vi "Find Average Center.vi"(7 "Tray Number":i32, 9 "XYZTheta":dbl[](array[numeric]), 11 "Gantry In":refnum<k24>) -> (1 "XYZTheta Centers":dbl[][](array[numeric]), 3 "Gantry Out":refnum<k24>)   [LabVIEW 2021, in "Assembly Tray.lvclass"]
uses:
  Assembly Tray.lvclass
  Controller/Camera/Machine Vision.ctl
  C:/Program Files (x86)/Aerotech/A3200/LabVIEW/2010/Bin/Aerotech.A3200.dll
  Program Files (x86)/Aerotech/A3200/LabVIEW/2010/Bin/Aerotech.A3200.dll
  Find Tray.ctl
  Controller/Camera/Camera settings.ctl
  Controller/Camera/Image processing.ctl
  Controller/Camera/Material.ctl
  Controller/Camera/Camera.lvclass
  Controller/Motion/A3200/A3200.lvclass
  Controller/Motion/Motion.lvclass
panel:
  out "Syringe Area Recorded":bool
  out "All fiducials recorded":bool
  out "XY Graph":cluster{"X":dbl, "Y":dbl}[](graph)
  in  "Go to P6":bool
  in  "Go to P5":bool
  out "P5 XY":dbl[](array[numeric])
  out "P6 XY":dbl[](array[numeric])
  in  "Record P6":bool
  in  "Record P5":bool
  in  "Focus step size":dbl format="%#_13g"
  in  "number of focus steps":i32
  in  "Focus":bool
  out "Average Strength":dbl
  in  "Material":T1
  in  "Image processing":T2={"Brightness"=128.0, "Contrast"=45.0, "Gamma"=1.0471123} {"Brightness" scale=0.0..400.0; "Contrast" scale=0.0..90.0; "Gamma" scale=0.005..5.0}
  in  "Camera settings":T3={"Gamma"=1.6, "Gain"=0, "Sharpness"=0, "Contrast"=0.0, "Exposure"=0.0078125} {"Exposure" min=0.000244140625 max=0.5 scale=0.0002..0.5; "Contrast" min=0.0 max=1.0 scale=0.001..1.0; "Sharpness" min=0 max=2 step=1 scale=0.0..2.0; "Gain" min=0 max=100 step=1 scale=0.1..100.0; "Gamma" min=0.01 max=10.0 scale=0.01..10.0}
  in  "Override presets":bool
  out "Center":dbl[](array[numeric])
  out "Syringe Area":dbl[](array[numeric])
  in  "Go to Syringe Area":bool
  in  "Record Syringe Area":bool
  in  "Carrier Tray":T4
  in  "Position":bool=TRUE
  in  "Go to Center":bool
  in  "Joystick":bool
  in  "Record P2":bool
  in  "Record P3":bool
  in  "Record P1":bool
  in  "Record P4":bool
  out "P3 XY":dbl[](array[numeric])
  out "P4 XY":dbl[](array[numeric])
  out "P2 XY":dbl[](array[numeric])
  out "P1 XY":dbl[](array[numeric])
  in  "Go to P1":bool
  in  "Go to P2":bool
  in  "Go to P3":bool
  in  "Go to P4":bool
  out "Gantry":dbl[](array[numeric])
  out "Sum":dbl[](array[numeric])
  in  "Stop Program":bool
  out "Image":T5(plugin-control)
  out "Camera":dbl[](array[numeric])
  in  "Machine Vision":T6
  # "1"
  # "2"
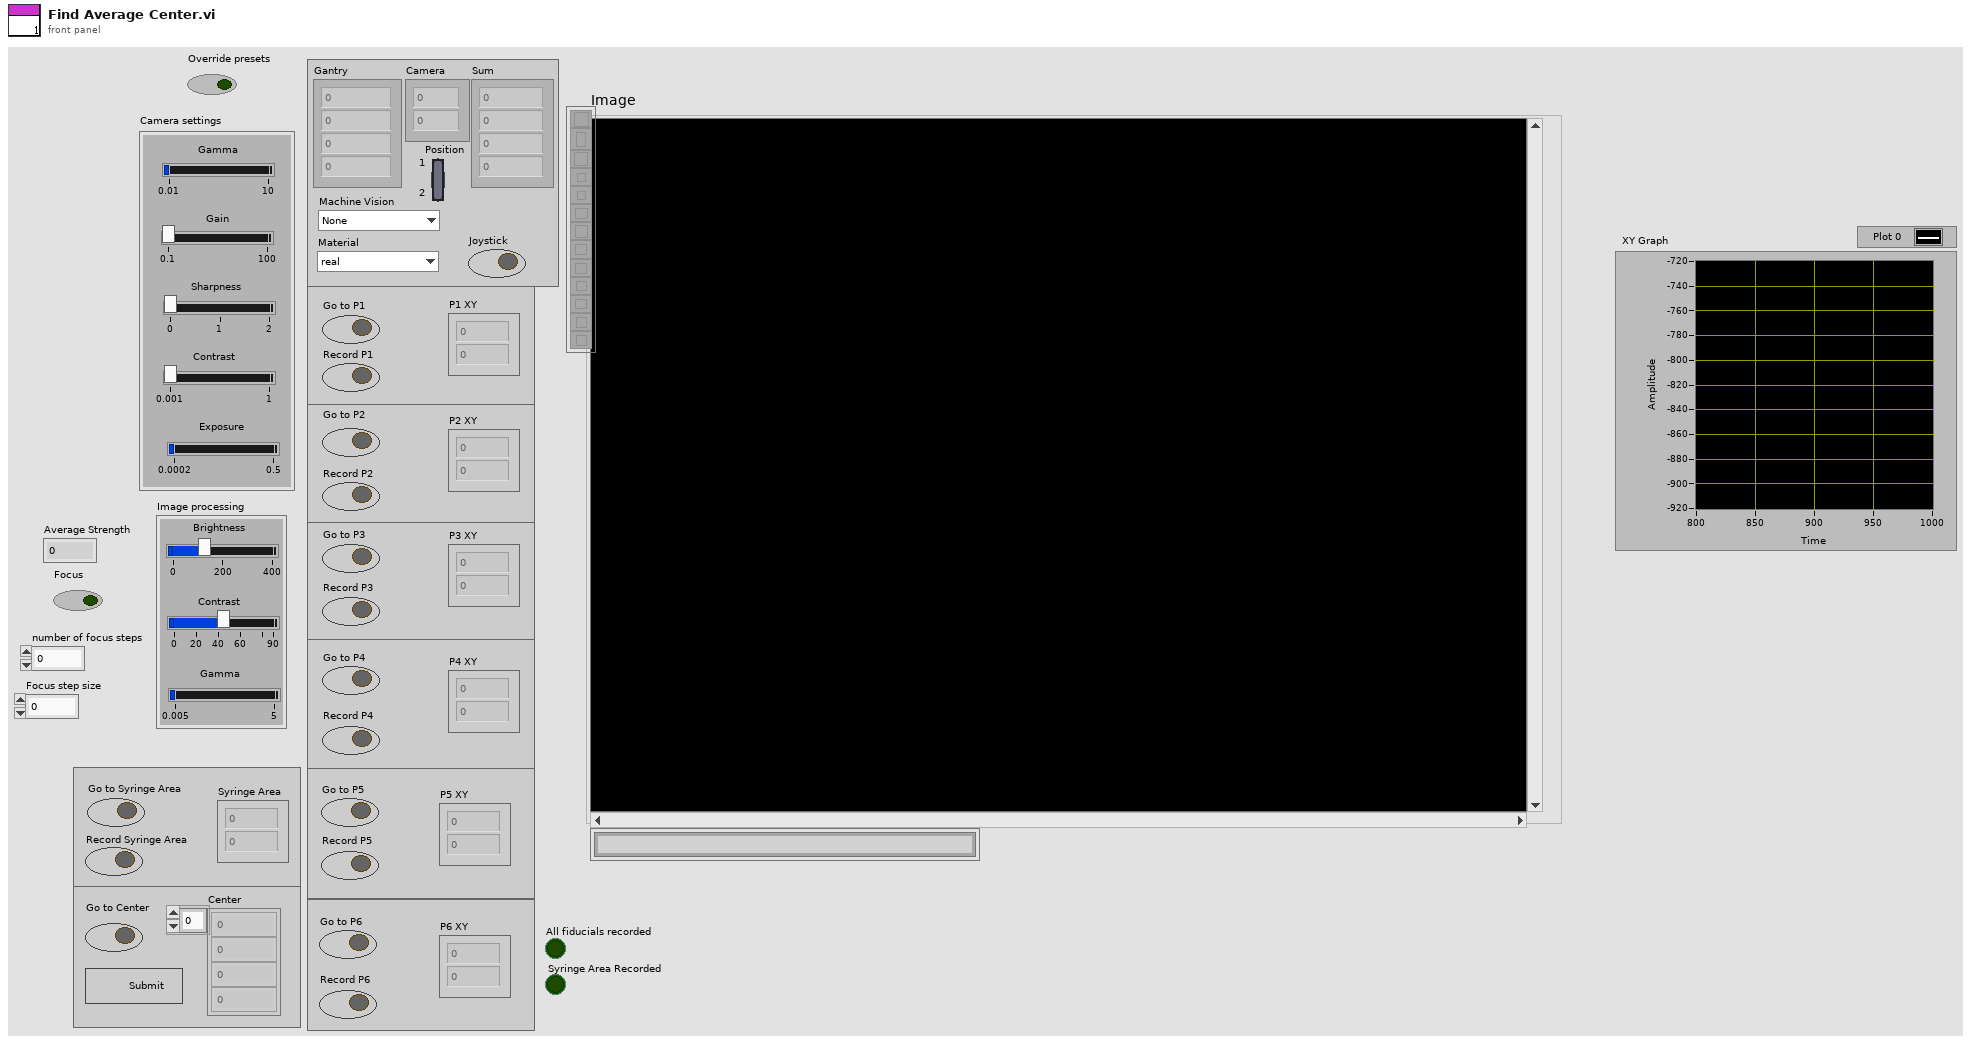
[diagram p1: front panel]
types:
  T1 = typedef "Camera.lvclass/Material.ctl" = enum16{"real", "dummy", "PETG"}
  T2 = typedef "Camera.lvclass/Image processing.ctl" = cluster{"Brightness":sgl, "Contrast":sgl, "Gamma":sgl}
  T3 = typedef "Camera.lvclass/Camera settings.ctl" = cluster{"Gamma":dbl, "Gain":i64, "Sharpness":i64, "Contrast":dbl, "Exposure":dbl}
  T4 = typedef "Assembly Tray.lvclass/Find Tray.ctl" = cluster{"Gantry Fiducials":dbl[], "Relative Coordinates":dbl[][], "Camera Fiducials":dbl[][], "XYZTheta Centers":dbl[][], "Workspace Center":dbl[], "Syringe Relative Coordinates":dbl[], "Gantry Region":dbl, "Fiducials":path, "New Fiducials":dbl[][], "Past Fiducials":dbl[][], "XYZTheta":dbl[], "Position":dbl}
  T5 = typedef "IMAQ Image.ctl" = refnum<image>
  T6 = typedef "Camera.lvclass/Machine Vision.ctl" = enum16{"None", "Tray Fiducials", "Sensor Fiducials", "HPK Silicon", "Partial Hexaboard", "Partial Hexaboard Test", "100um dot", "Hexaboard", "Corner (TL, BR)", "Corner (BL, TR)", "V3 Sensor Cross", "V3 Sensor Circle"}
  T7 = typedef "File Paths.ctl" = cluster{"Glue Pattern Folder":path, "Carrier Tray Folder":path, "Pick Up Tool Fixture Folder":path, "Components Folder":path, "Bellows Tool Offset.txt":path, "Pick Up Tool Offset.txt":path, "Dispense Tip Offset.txt":path, "Log Files":path, "Gantry Assembly Map.txt":path, "Syringe and offset map.txt":path}
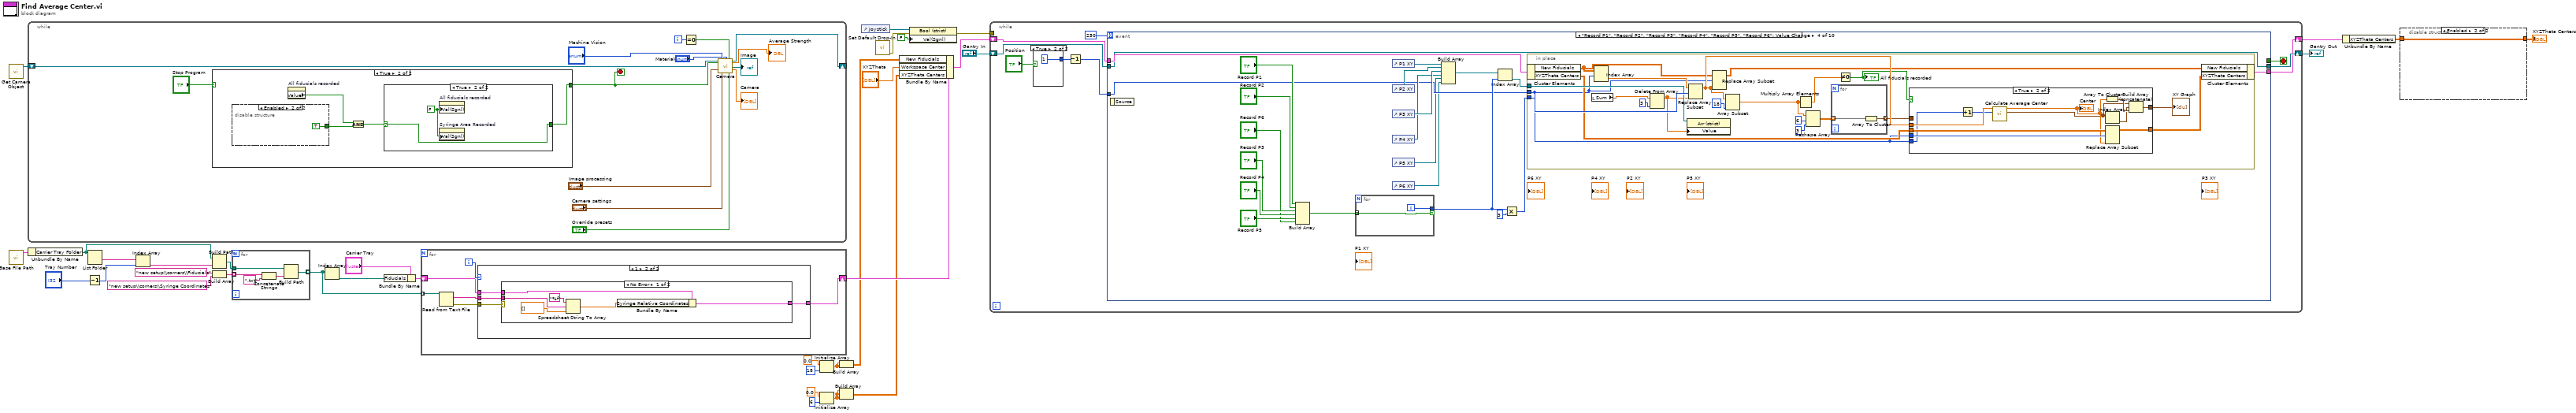
[diagram p0: block diagram]
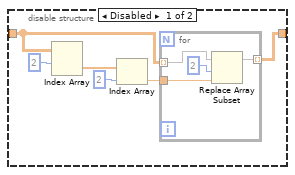
[diagram p2: hidden frame]
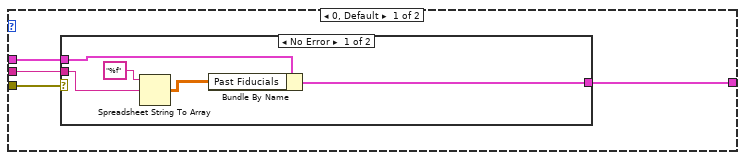
[diagram p3: hidden frame]
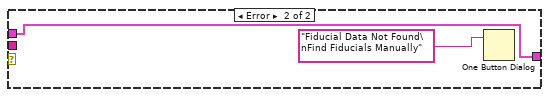
[diagram p4: hidden frame]
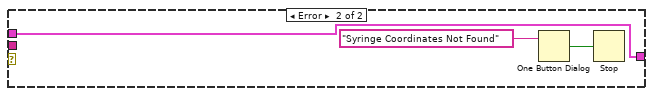
[diagram p5: hidden frame]
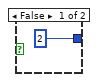
[diagram p6: hidden frame]
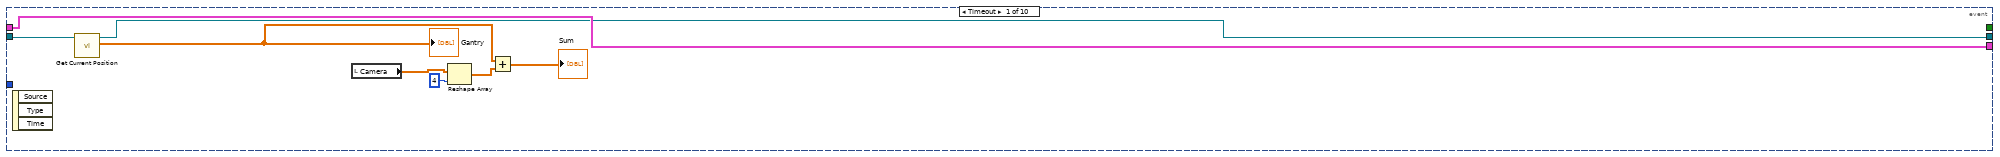
[diagram p7: hidden frame]
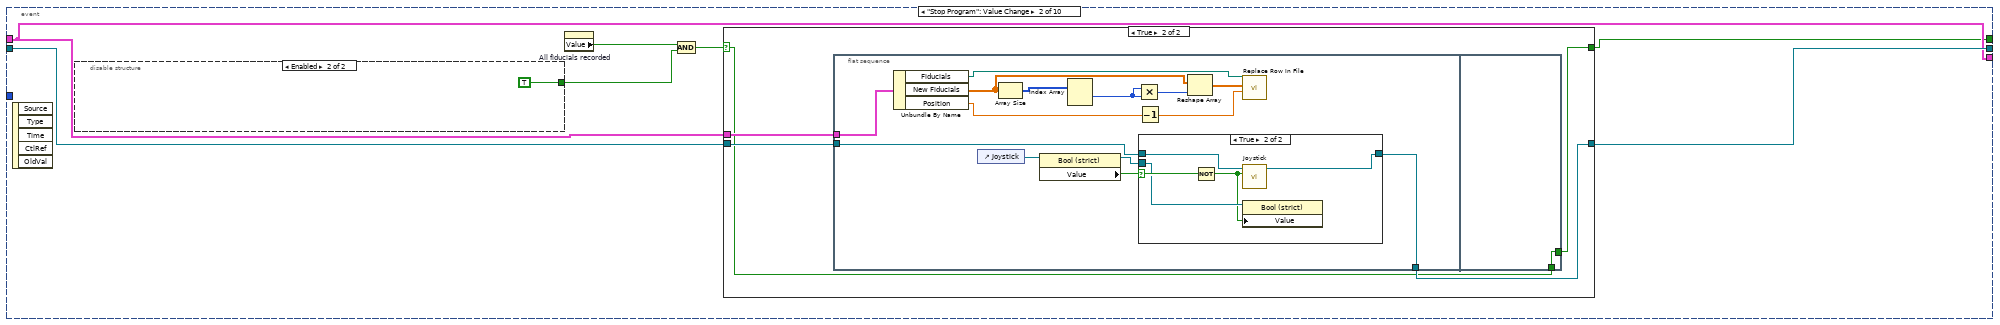
[diagram p8: hidden frame]
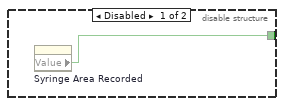
[diagram p9: hidden frame]
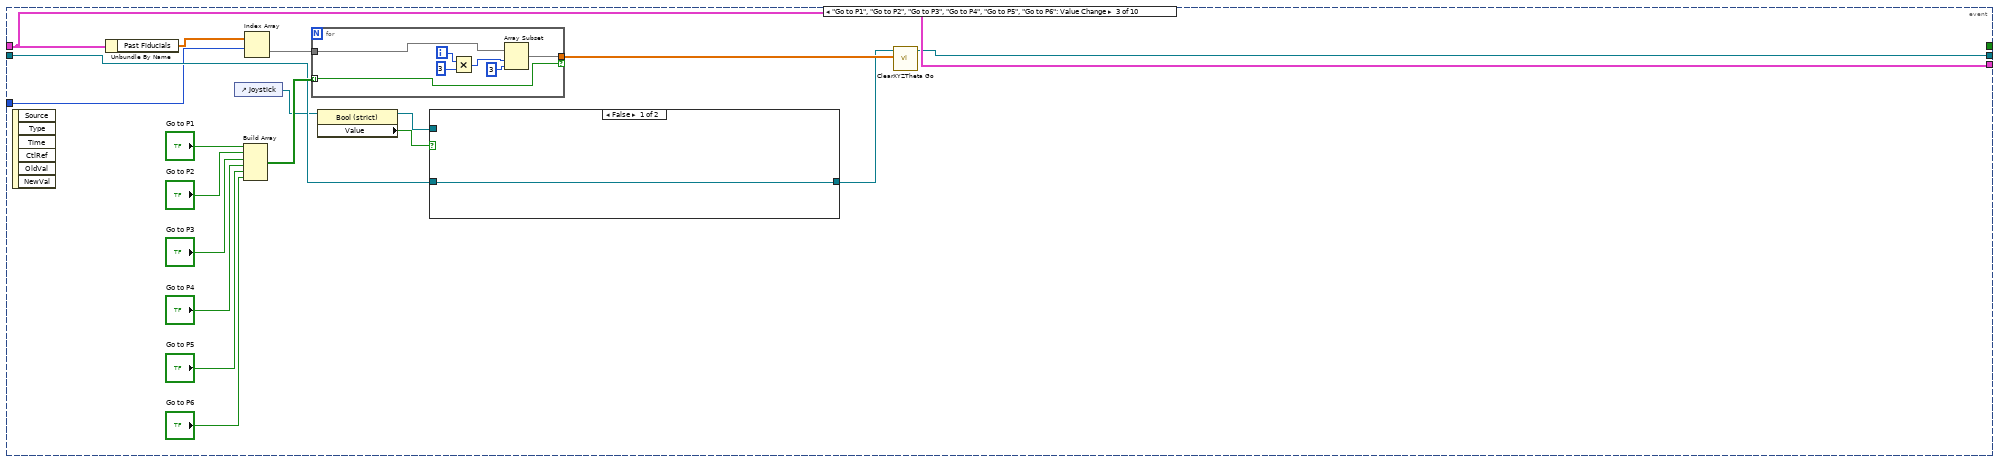
[diagram p12: hidden frame]
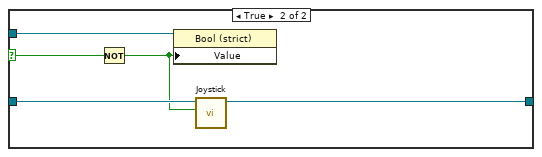
[diagram p13: hidden frame]
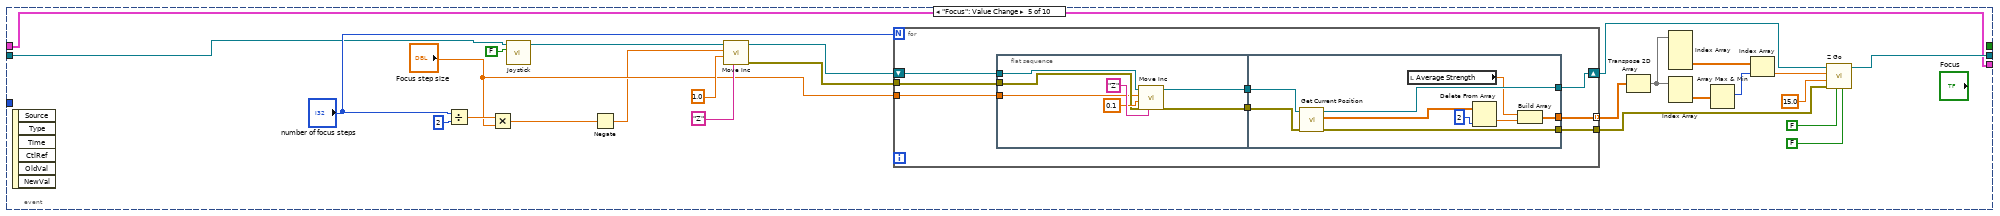
[diagram p15: hidden frame]
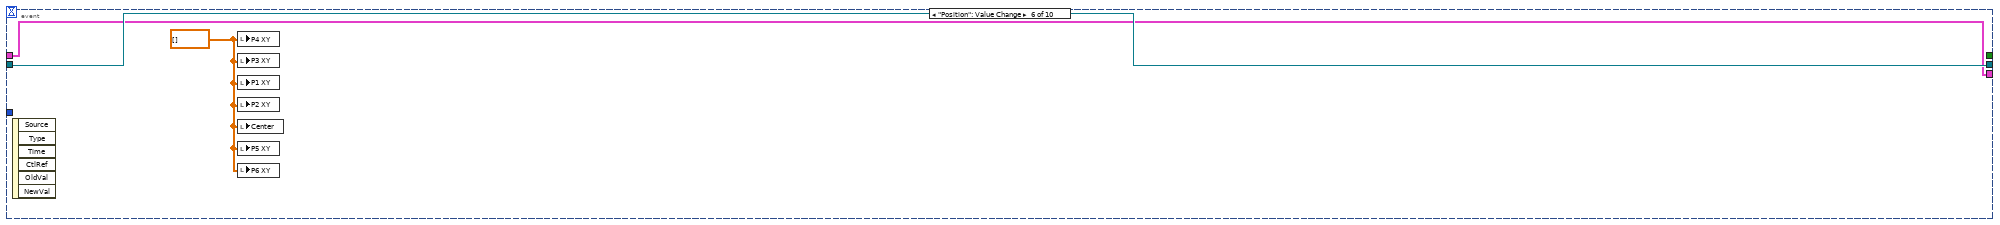
[diagram p16: hidden frame]
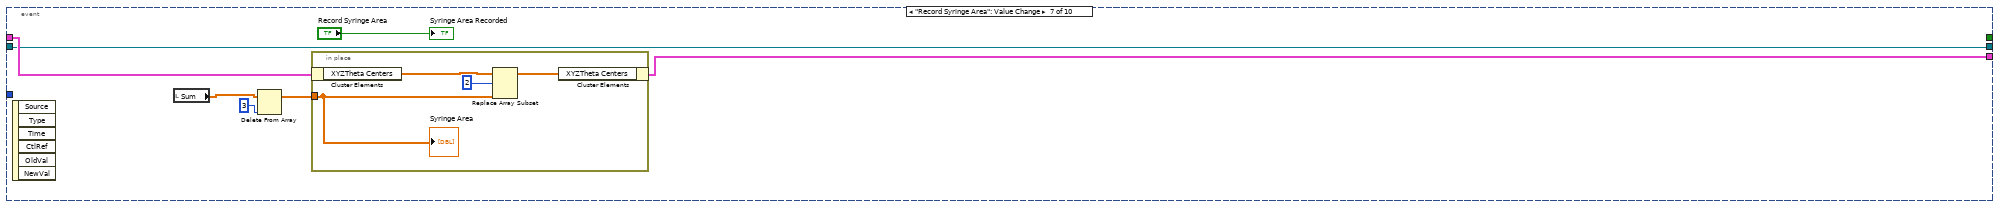
[diagram p17: hidden frame]
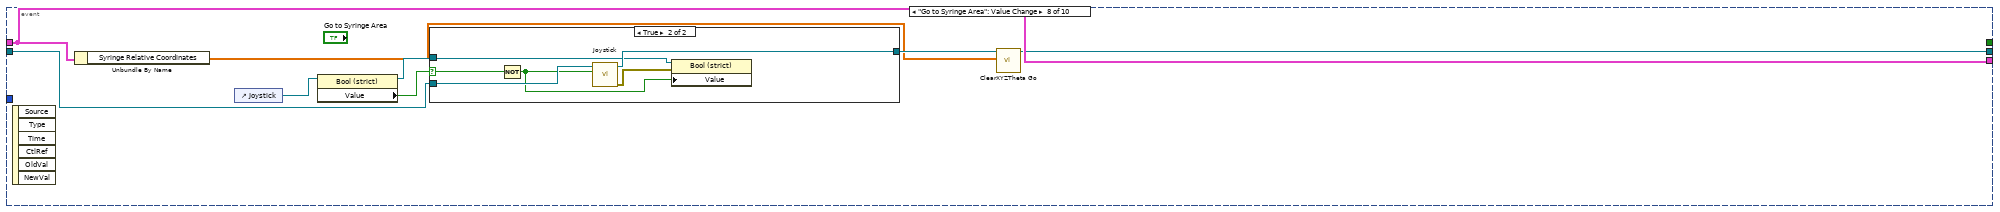
[diagram p18: hidden frame]
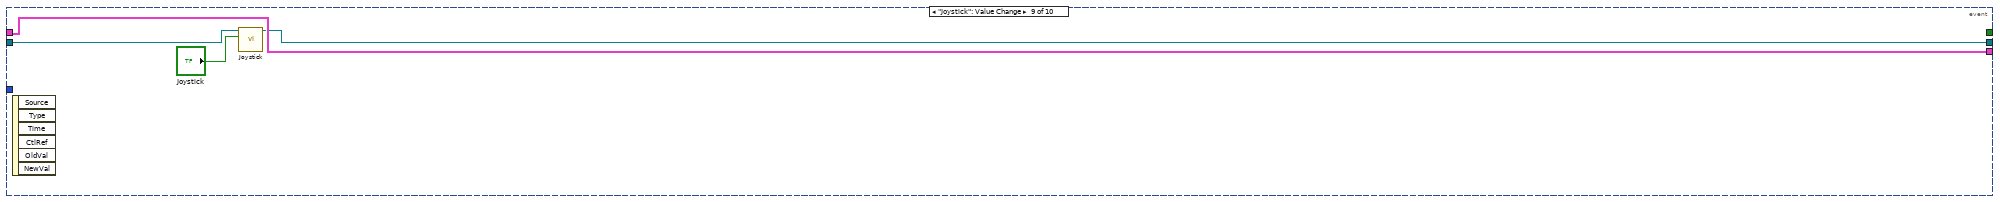
[diagram p20: hidden frame]
diagram:
  n1 = call "Get Camera Object.vi"() -> ("Camera out"=w3:refnum<class "Camera.lvclass">)  [unwired: 10 in, 1 out]
  n2 = call "Base File Path.vi"() -> ("Paths Out"=w19:T7)  [unwired: 11 in]
  n3 = while {
    shift-right: [w45] -> _
    shift-left: w3 -> [w49]
    i -> [w41]
    stop <- w36 stop-if-true
    n4 = case shown="True" "Stop Program" {
      selector: "Stop Program" -> [w50 _]
      tunnel: [w50 w51] -> w36
      frame False {
      }
      frame True {
        n5 = disable-structure shown="Enabled" {
          disable-tunnel: [w55 TRUE ("Value")] -> w53
          frame Disabled {
            n6 = property on="Syringe Area Recorded" class="Bool (strict)"() -> ("Value"=w55:bool)  [unwired: 2 in, 2 out]
          }
          frame Enabled {
          }
        }
        n7 = property on="All fiducials recorded" class="Bool (strict)"() -> ("Value"=w54:bool)  [unwired: 2 in, 2 out]
        n8 = And(x=w54, y=w53) -> (x .and. y?=w52:bool)
        n9 = case shown="True" w52 {
          selector: w52 -> [w58 w59]
          tunnel: [w58 w59] -> w51
          frame False {
            n10 = One Button Dialog(message="At least one fiducial or syringe loading area not recorded.") -> ()  [unwired: 1 in, 1 out]
          }
          frame True {
            w60 = FALSE ("Value (Signaling)")
            n11 = property on="All fiducials recorded" class="Bool (strict)"("Val(Sgnl)"=w60) -> ()  [unwired: 2 in, 2 out]
            n12 = property on="Syringe Area Recorded" class="Bool (strict)"("Val(Sgnl)"=w60) -> ()  [unwired: 2 in, 2 out]
          }
        }
      }
    }
    n13 = Equal To 0?(x=w41) -> (x = 0?=w40:bool)
    n14 = call "Camera.vi"("Camera in"=w49, "Stop"=w36, "BCG Image Processing"="Image processing", "Machine Vision"="Machine Vision", "Camera settings"="Camera settings", "Material"="Material", "Loop 0"=w40, "Override presets"="Override presets") -> ("Camera out"=w45:refnum<class "Camera.lvclass">, "Average Strength"=→"Average Strength":dbl, "Image"=→"Image":T5, "Camera"=→"Camera":dbl[])  [unwired: 5 in, 3 out]
  }
  n15 = Unbundle By Name(w19) -> ("Carrier Tray Folder"=w17:path)
  n16 = Decrement(x="Tray Number") -> (x-1=w18:i32)
  n17 = List Folder(path=w17) -> (folder names=w21:string[])  [unwired: 3 in, 3 out]
  n18 = Index Array(array=w21, index=w18) -> (element=w20:string)
  n19 = Build Path(base path=w17, name or relative path=w20) -> (appended path=w23:path)
  n20 = Build Array("new setup\\corners\\Fiducials" ("format string"), "new setup\\corners\\Syringe Coordinates" ("element")) -> (w22:string[])
  n21 = for {
    tunnel: w22 -> [w63] mode=indexing
    tunnel: w23 -> [w65]
    tunnel: [w64] -> w16 mode=indexing
    n22 = Concatenate Strings(w63, ".txt" ("string")) -> (w61:string)
    n23 = Build Path(base path=w65, name or relative path=w61) -> (appended path=w64:path)
  }
  n24 = Index Array(array=w16) -> (element=w2:path)  [unwired: 1 in]
  n25 = Bundle By Name(cluster="Carrier Tray", "Fiducials"=w2) -> (w25:T4)
  n26 = for {
    tunnel: w16 -> [w70] mode=indexing
    shift-right: [w66] -> w13
    shift-left: w25 -> [w67]
    i -> [w68]
    n27 = Read from Text File(file (use dialog)=w70) -> (text=w71:string, error out=w69:errorcluster)  [unwired: 3 in, 2 out]
    n28 = case shown="1" w68 {
      tunnel: w71 -> [w75 w84]
      tunnel: w69 -> [w74 w85]
      tunnel: w67 -> [w73 w86]
      tunnel: [w72 w83] -> w66
      frame 0, Default {
        n29 = case shown="No Error" w74 {
          tunnel: w75 -> [w79 _]
          tunnel: w73 -> [w77 w81]
          tunnel: [w78 w81] -> w72
          frame No Error {
            n30 = Spreadsheet String To Array(format string="%f", spreadsheet string=w79) -> (array=w76:dbl[][])  [unwired: 2 in]
            n31 = Bundle By Name(cluster=w77, "Past Fiducials"=w76) -> (w78:T4)
          }
          frame Error {
            n32 = One Button Dialog(message="Fiducial Data Not Found\nFind Fiducials Manually") -> ()  [unwired: 1 in, 1 out]
          }
        }
      }
      frame 1 {
        n33 = case shown="No Error" w85 {
          tunnel: w84 -> [w90 _]
          tunnel: [w88 w93] -> w83
          tunnel: w86 -> [w89 w93]
          frame No Error {
            n34 = Spreadsheet String To Array(format string="%f", spreadsheet string=w90, array type (2D Dbl)=dbl[] []) -> (array=w87:dbl[])  [unwired: 1 in]
            n35 = Bundle By Name(cluster=w89, "Syringe Relative Coordinates"=w87) -> (w88:T4)
          }
          frame Error {
            n36 = One Button Dialog(message="Syringe Coordinates Not Found") -> (true=w94:bool)  [unwired: 1 in]
            n37 = Stop(stop? (T)=w94) -> ()
          }
        }
      }
    }
  }
  n38 = Initialize Array(0.0 ("element"), 18 ("dimension size")) -> (w11:dbl[])
  n39 = Initialize Array(0.0 ("element"), 6 ("dimension size")) -> (w7:dbl[])
  n40 = Build Array(w11, w11) -> (w1:dbl[][])
  n41 = Build Array(w7, w7, w7) -> (w6:dbl[][])
  n42 = control-ref of="Joystick"() -> (w34:refnum<vi>)
  n43 = call "Set Default Drop-In.vi"() -> ("error out"=w28:errorcluster)  [unwired: 11 in]
  n44 = Bundle By Name(cluster=w13, "New Fiducials"=w1, "Workspace Center"="XYZTheta", "XYZTheta Centers"=w6) -> (w35:T4)
  n45 = property class="Bool (strict)"(reference=w34, error in=w28, "Val(Sgnl)"=FALSE) -> (error out=w32:errorcluster)  [unwired: 1 out]
  n46 = while {
    shift-right: [w97] -> w10
    shift-left: w35 -> [w104]
    tunnel: w32 -> [_]
    shift-right: [w101] -> w26
    shift-left: "Gantry In" -> [w102]
    stop <- w96 stop-if-true
    n47 = case shown="True" "Position" {
      tunnel: [2 1] -> w98
      frame False {
      }
      frame True {
      }
    }
    n48 = Decrement(x=w98) -> (x-1=w100:i32)
    n49 = event shown="[3] \"Record P1\", \"Record P2\", \"Record P3\", \"Record P4\", \"Record P5\", \"Record P6\": Value Change" {
      selector: _ -> [_ _ _ _ _ _ _ _ _ _]
      dyn-events: _ -> [_ _ _ _ _ _ _ _ _ _]
      timeout: 250 -> [_ _ _ _ _ _ _ _ _ _]
      tunnel: w104 -> [w113 w120 w163 w190 w245 w294 w302 w314 w325 w335]
      tunnel: [w113 w120 w163 w204 w245 w294 w301 w314 w325 w335] -> w97
      tunnel: w102 -> [w109 w119 w160 w183 w247 w295 w300 w313 w324 w331]
      tunnel: [w108 w121 w157 w183 w246 w295 w300 w308 w322 w329] -> w101
      tunnel: w100 -> [_ _ w154 w189 _ _ _ _ _ w327]
      tunnel: [_ w115 _ _ _ _ _ _ _ _] -> w96
      event Timeout {
        n50 = event-data() -> ()  [unwired: 1 in, 3 out]
        n51 = call "Get Current Position.vi"("Gantry In"=w109) -> ("XYZTheta Out"=w107:dbl[], "Gantry Out"=w108:refnum<k24>)  [unwired: 8 in, 1 out]
        "Gantry" <- w107
        n52 = local read "Camera"() -> (w112:dbl[])
        n53 = Reshape Array(w112, 4 ("dimension size")) -> (w110:dbl[])
        n54 = Add(x=w107, y=w110) -> (x+y=→"Sum":dbl[])
      }
      event "Stop Program": Value Change {
        n55 = event-data() -> ()  [unwired: 1 in, 5 out]
        n56 = disable-structure shown="Enabled" {
          disable-tunnel: [w122 TRUE ("Value")] -> w117
          frame Disabled {
            n57 = property on="Syringe Area Recorded" class="Bool (strict)"() -> ("Value"=w122:bool)  [unwired: 2 in, 2 out]
          }
          frame Enabled {
          }
        }
        n58 = property on="All fiducials recorded" class="Bool (strict)"() -> ("Value"=w118:bool)  [unwired: 2 in, 2 out]
        n59 = And(x=w118, y=w117) -> (x .and. y?=w116:bool)
        n60 = case shown="True" w116 {
          selector: w116 -> [w124 w127]
          tunnel: [w125 w130] -> w121
          tunnel: w120 -> [_ w129]
          tunnel: w119 -> [w125 w128]
          tunnel: [w124 w126] -> w115
          frame False {
          }
          frame True {
            n61 = flat-sequence {
              tunnel: [w144] -> w130
              tunnel: w129 -> [w135]
              tunnel: w128 -> [w131]
              tunnel: w127 -> [w151]
              tunnel: [w151] -> w126
              frame #0 {
                n62 = Unbundle By Name(w135) -> ("Fiducials"=w132:path, "New Fiducials"=w137:dbl[][], "Position"=w136:dbl)
                n63 = control-ref of="Joystick"() -> (w143:refnum<vi>)
                n64 = Array Size(array=w137) -> (size(s)=w138:i32[])
                n65 = property class="Bool (strict)"(reference=w143) -> (reference out=w142:refnum<vi>, "Value"=w141:bool)  [unwired: 1 in, 1 out]
                n66 = Index Array(array=w138) -> (element #1=w139:i32)  [unwired: 2 in, 1 out]
                n67 = Multiply(x=w139, y=w139) -> (x*y=w140:i32)
                n68 = Decrement(x=w136) -> (x-1=w133:dbl)
                n69 = case shown="True" w141 {
                  selector: w141 -> [_ w150]
                  tunnel: [w145 w148] -> w144
                  tunnel: w142 -> [_ w149]
                  tunnel: w131 -> [w145 w146]
                  frame False {
                  }
                  frame True {
                    n70 = Not(x=w150) -> (.not. x?=w147:bool)
                    n71 = call "Joystick.vi"("Joystick"=w147, "Gantry In"=w146) -> ("Gantry Out"=w148:refnum<k24>)  [unwired: 8 in, 1 out]
                    n72 = property class="Bool (strict)"(reference=w149, "Value"=w147) -> ()  [unwired: 1 in, 2 out]
                  }
                }
                n73 = Reshape Array(w137, w140) -> (w134:dbl[])
                n74 = call "Replace Row In File.vi"("Index"=w133, "Insert Array"=w134, "Path"=w132) -> ()  [unwired: 8 in, 1 out]
              }
              frame #1 {
              }
            }
          }
        }
      }
      event "Go to P1", "Go to P2", "Go to P3", "Go to P4", "Go to P5", "Go to P6": Value Change {
        n75 = event-data() -> ()  [unwired: 1 in, 6 out]
        n76 = Unbundle By Name(w163) -> ("Past Fiducials"=w156:dbl[][])
        n77 = control-ref of="Joystick"() -> (w158:refnum<vi>)
        n78 = Build Array("Go to P1", "Go to P2", "Go to P3", "Go to P4", "Go to P5", "Go to P6") -> (w165:bool[])
        n79 = Index Array(array=w156, index (row)=w154) -> (element=w155:dbl[])  [unwired: 1 in]
        n80 = for {
          tunnel: w165 -> [w182] mode=indexing
          tunnel: w155 -> [w181]
          tunnel: [w176] -> w164 if=w182
          i -> [w179]
          n81 = Multiply(x=w179, y=3) -> (x*y=w177:i32)
          n82 = Array Subset(array=w181, index=w177, length=3) -> (w176:dbl[])
        }
        n83 = property class="Bool (strict)"(reference=w158) -> (reference out=w161:refnum<vi>, "Value"=w162:bool)  [unwired: 1 in, 1 out]
        n84 = case shown="False" w162 {
          selector: w162 -> [_ w175]
          tunnel: w160 -> [w170 w173]
          tunnel: [w170 w171] -> w159
          tunnel: w161 -> [_ w174]
          frame False {
          }
          frame True {
            n85 = Not(x=w175) -> (.not. x?=w172:bool)
            n86 = property class="Bool (strict)"(reference=w174, "Value"=w172) -> ()  [unwired: 1 in, 2 out]
            n87 = call "Joystick.vi"("Joystick"=w172, "Gantry In"=w173) -> ("Gantry Out"=w171:refnum<k24>)  [unwired: 8 in, 1 out]
          }
        }
        n88 = call "ClearXYZTheta Go.vi"("XYZTheta In"=w164, "Gantry In"=w159) -> ("Gantry Out"=w157:refnum<k24>)  [unwired: 7 in, 2 out]
      }
      event "Record P1", "Record P2", "Record P3", "Record P4", "Record P5", "Record P6": Value Change {
        n89 = event-data() -> ()  [unwired: 1 in, 1 out]
        n90 = Build Array("Record P1", "Record P2", "Record P3", "Record P4", "Record P5", "Record P6") -> (w199:bool[])
        n91 = for {
          tunnel: w199 -> [w205] mode=indexing
          tunnel: [w206] -> w192 if=w205
          i -> [w206]
        }
        n92 = control-ref of="P1 XY"() -> (w198:refnum<vi>)
        n93 = control-ref of="P2 XY"() -> (w197:refnum<vi>)
        n94 = control-ref of="P3 XY"() -> (w196:refnum<vi>)
        n95 = control-ref of="P4 XY"() -> (w195:refnum<vi>)
        n96 = control-ref of="P5 XY"() -> (w186:refnum<vi>)
        n97 = control-ref of="P6 XY"() -> (w185:refnum<vi>)
        n98 = Build Array(w198, w197, w196, w195, w186, w185) -> (w194:refnum<vi>[])
        n99 = Index Array(array=w194, index=w192) -> (element=w193:refnum<vi>)
        n100 = Multiply(x=w192, y=3) -> (x*y=w184:i32)
        n101 = in-place {
          in-place-border: w184 -> [w227]
          in-place-border: w193 -> [w226]
          in-place-border: w189 -> [w207]
          n102 = in-place-cluster #1(w190) -> ("New Fiducials"=w219:dbl[][], "XYZTheta Centers"=w221:dbl[][])
          n103 = local read "Sum"() -> (w218:dbl[])
          n104 = Index Array(array=w219, index (row)=w207) -> (element=w222:dbl[])  [unwired: 1 in]
          n105 = Delete From Array(array=w218, index=3) -> (array with subset deleted=w216:dbl[])  [unwired: 1 in, 1 out]
          n106 = property class="Arr (strict)"(reference=w226, "Value"=w216) -> ()  [unwired: 1 in, 2 out]
          n107 = Replace Array Subset(array=w222, new element=w216, index=w227) -> (w225:dbl[])
          n108 = Replace Array Subset "Replace Array Subset"(array=w219, new element=w225, index (row)=w207) -> (w208:dbl[][])  [unwired: 1 in]
          n109 = Array Subset(array=w225, length=18) -> (w215:dbl[])  [unwired: 1 in]
          n110 = Multiply Array Elements(1:w215) -> (0:w223:dbl)
          n111 = Reshape Array(w215, 6 ("dimension size"), 3 ("dimension size")) -> (w212:dbl[][])
          n112 = for {
            tunnel: [w229] -> w210 mode=indexing
            tunnel: w212 -> [w228] mode=indexing
            n113 = Array To Cluster(array=w228) -> (cluster=w229:cluster{"[0]":dbl, "[1]":dbl})
          }
          n114 = Not Equal To 0?(x=w223) -> (x != 0?=w211:bool)
          "All fiducials recorded" <- w211
          n115 = case shown="True" w211 {
            tunnel: w225 -> [_ w240]
            tunnel: w221 -> [w231 w242]
            tunnel: w207 -> [_ w239]
            tunnel: [w231 w241] -> w220
            tunnel: w207 -> [_ w237]
            tunnel: w210 -> [w230 _]
            tunnel: [w230 w238] -> w209
            frame False {
            }
            frame True {
              n116 = Increment(x=w237) -> (x+1=w236:i32)
              n117 = call "Calculate Average Center.vi"("Position"=w236, "Gantry Fiducials"=w240) -> ("Array"=w233:cluster{"X":sgl, "Y":sgl}[], "XYZTheta"=w235:dbl[])  [unwired: 8 in]
              "Center" <- w235
              n118 = Array To Cluster(array=w235) -> (cluster=w234:cluster{"XYZTheta[0]":dbl, "XYZTheta[1]":dbl})
              n119 = Index Array(array=w233) -> (element=w232:cluster{"X":sgl, "Y":sgl})  [unwired: 1 in]
              n120 = Replace Array Subset(array=w242, new element=w235, index (row)=w239) -> (w241:dbl[][])  [unwired: 1 in]
              n121 = Build Array (concatenate)(w233, w232, w234) -> (w238:cluster{"XYZTheta[0]":dbl, "XYZTheta[1]":dbl}[])
            }
          }
          "XY Graph" <- w209
          n122 = in-place-cluster #1("New Fiducials"=w208, "XYZTheta Centers"=w220) -> (w204:T4)
        }
      }
      event "Focus": Value Change {
        n123 = event-data() -> ()  [unwired: 1 in, 6 out]
        n124 = Divide(x="number of focus steps", y=2) -> (x/y=w251:dbl)
        n125 = Multiply(x=w251, y="Focus step size") -> (x*y=w249:dbl)
        n126 = call "Joystick.vi"("Joystick"=FALSE, "Gantry In"=w247) -> ("Gantry Out"=w254:refnum<k24>)  [unwired: 8 in, 1 out]
        n127 = Negate(x=w249) -> (-x=w248:dbl)
        n128 = call "Move Inc.vi"("Axis"="Z", "Speed"=1.0, "Distance"=w248, "Gantry In"=w254) -> ("error out"=w257:errorcluster, "Gantry Out"=w268:refnum<k24>)  [unwired: 6 in]
        n129 = for {
          N: "number of focus steps" -> [_]
          tunnel: [w273] -> w264 mode=indexing
          tunnel: w257 -> [w272]
          tunnel: [w270] -> w256
          shift-right: [w274] -> w258
          shift-left: w268 -> [w276]
          tunnel: "Focus step size" -> [w269]
          n130 = flat-sequence {
            tunnel: w276 -> [w281]
            tunnel: [w280] -> w275
            tunnel: w272 -> [w279]
            tunnel: [w278] -> w271
            tunnel: w269 -> [w277]
            tunnel: w275 -> [w292]
            tunnel: [w291] -> w274
            tunnel: [w290] -> w273
            tunnel: w271 -> [w286]
            tunnel: [w285] -> w270
            frame #0 {
              n131 = call "Move Inc.vi"("Axis"="Z", "error in (no error)"=w279, "Speed"=0.1, "Distance"=w277, "Gantry In"=w281) -> ("error out"=w278:errorcluster, "Gantry Out"=w280:refnum<k24>)  [unwired: 5 in]
            }
            frame #1 {
              n132 = call "Get Current Position.vi"("error in (no error)"=w286, "Gantry In"=w292) -> ("error out"=w285:errorcluster, "XYZTheta Out"=w289:dbl[], "Gantry Out"=w291:refnum<k24>)  [unwired: 7 in]
              n133 = local read "Average Strength"() -> (w284:dbl)
              n134 = Delete From Array(array=w289, index=2) -> (deleted portion=w287:dbl)  [unwired: 1 in, 1 out]
              n135 = Build Array(w284, w287) -> (w290:dbl[])
            }
          }
        }
        n136 = Transpose 2D Array(2D array=w264) -> (transposed array=w263:dbl[][])
        n137 = Index Array(array=w263) -> (element #2=w262:dbl[])  [unwired: 4 in, 1 out]
        n138 = Index Array(array=w263) -> (element=w265:dbl[])  [unwired: 2 in]
        n139 = Array Max & Min(array=w265) -> (max index (indices)=w261:i32)  [unwired: 3 out]
        n140 = Index Array(array=w262, index=w261) -> (element=w260:dbl)
        n141 = call "Z Go.vi"("Increment"=FALSE, "Return Immediately"=FALSE, "error in (no error)"=w256, "Speed In"=15.0 ("Speed"), "Position In"=w260, "Gantry In"=w258) -> ("Gantry Out"=w246:refnum<k24>)  [unwired: 2 in, 3 out]
      }
      event "Position": Value Change {
        w293 = dbl[] [] ("TR XY")
        n142 = event-data() -> ()  [unwired: 1 in, 6 out]
        n143 = local write "P4 XY"(w293) -> ()
        n144 = local write "P3 XY"(w293) -> ()
        n145 = local write "P1 XY"(w293) -> ()
        n146 = local write "P2 XY"(w293) -> ()
        n147 = local write "Center"(w293) -> ()
        n148 = local write "P5 XY"(w293) -> ()
        n149 = local write "P6 XY"(w293) -> ()
      }
      event "Record Syringe Area": Value Change {
        n150 = event-data() -> ()  [unwired: 1 in, 6 out]
        n151 = local read "Sum"() -> (w299:dbl[])
        n152 = Delete From Array(array=w299, index=3) -> (array with subset deleted=w298:dbl[])  [unwired: 1 in, 1 out]
        n153 = in-place {
          in-place-border: w298 -> [w305]
          n154 = in-place-cluster #2(w302) -> ("XYZTheta Centers"=w306:dbl[][])
          n155 = Replace Array Subset(array=w306, new element=w305, index (row)=2) -> (w303:dbl[][])  [unwired: 1 in]
          n156 = in-place-cluster #2("XYZTheta Centers"=w303) -> (w301:T4)
          "Syringe Area" <- w305
        }
        "Syringe Area Recorded" <- "Record Syringe Area"
      }
      event "Go to Syringe Area": Value Change {
        n157 = event-data() -> ()  [unwired: 1 in, 6 out]
        n158 = Unbundle By Name(w314) -> ("Syringe Relative Coordinates"=w307:dbl[])
        n159 = control-ref of="Joystick"() -> (w312:refnum<vi>)
        n160 = property class="Bool (strict)"(reference=w312) -> (reference out=w310:refnum<vi>, "Value"=w311:bool)  [unwired: 1 in, 1 out]
        n161 = case shown="True" w311 {
          selector: w311 -> [_ w317]
          tunnel: [w315 w321] -> w309
          tunnel: w313 -> [w315 w320]
          tunnel: w310 -> [_ w319]
          frame False {
          }
          frame True {
            n162 = Not(x=w317) -> (.not. x?=w316:bool)
            n163 = call "Joystick.vi"("Joystick"=w316, "Gantry In"=w320) -> ("error out"=w318:errorcluster, "Gantry Out"=w321:refnum<k24>)  [unwired: 8 in]
            n164 = property class="Bool (strict)"(reference=w319, error in=w318, "Value"=w316) -> ()  [unwired: 2 out]
          }
        }
        n165 = call "ClearXYZTheta Go.vi"("XYZTheta In"=w307, "Gantry In"=w309) -> ("Gantry Out"=w308:refnum<k24>)  [unwired: 7 in, 2 out]
      }
      event "Joystick": Value Change {
        n166 = event-data() -> ()  [unwired: 1 in, 6 out]
        n167 = call "Joystick.vi"("Joystick"="Joystick", "Gantry In"=w324) -> ("Gantry Out"=w322:refnum<k24>)  [unwired: 8 in, 1 out]
      }
      event "Go to Center": Value Change {
        n168 = event-data() -> ()  [unwired: 1 in, 6 out]
        n169 = Unbundle By Name(w335) -> ("XYZTheta Centers"=w328:dbl[][])
        n170 = control-ref of="Joystick"() -> (w332:refnum<vi>)
        n171 = Index Array(array=w328, index (row)=w327) -> (element=w326:dbl[])  [unwired: 1 in]
        n172 = property class="Bool (strict)"(reference=w332) -> (reference out=w333:refnum<vi>, "Value"=w334:bool)  [unwired: 1 in, 1 out]
        n173 = case shown="True" w334 {
          selector: w334 -> [_ w342]
          tunnel: w331 -> [w336 w339]
          tunnel: [w336 w338] -> w330
          tunnel: w333 -> [_ w341]
          frame False {
          }
          frame True {
            n174 = Not(x=w342) -> (.not. x?=w337:bool)
            n175 = call "Joystick.vi"("Joystick"=w337, "Gantry In"=w339) -> ("error out"=w340:errorcluster, "Gantry Out"=w338:refnum<k24>)  [unwired: 8 in]
            n176 = property class="Bool (strict)"(reference=w341, error in=w340, "Value"=w337) -> ()  [unwired: 2 out]
          }
        }
        n177 = call "ClearXYZTheta Go.vi"("XYZTheta In"=w326, "Gantry In"=w330) -> ("Gantry Out"=w329:refnum<k24>)  [unwired: 7 in, 2 out]
      }
    }
  }
  "Gantry Out" <- w26
  n178 = Unbundle By Name(w10) -> ("XYZTheta Centers"=w5:dbl[][])
  n179 = disable-structure shown="Enabled" {
    disable-tunnel: w5 -> [w345 w353]
    disable-tunnel: [w343 w353] -> w4
    frame Disabled {
      n180 = Index Array(array=w345, index (row)=2) -> (element=w347:dbl[])  [unwired: 1 in]
      n181 = Index Array(array=w347, index=2) -> (element=w344:dbl)
      n182 = for {
        tunnel: w345 -> [w352] mode=indexing
        tunnel: w344 -> [w351]
        tunnel: [w350] -> w343 mode=indexing
        n183 = Replace Array Subset(array=w352, new element=w351, index=2) -> (w350:dbl[])
      }
    }
    frame Enabled {
    }
  }
  "XYZTheta Centers" <- w4
